vi "replaceTypeToken.vi"(8 "error in (no error)":errorcluster, 10 "Query In":string, 11 "Credit Transaction in":refnum<class "CreditTransaction.lvclass">) -> (0 "error out":errorcluster, 2 "Query Out":string, 3 "Credit Transaction out":refnum<class "CreditTransaction.lvclass">)   [LabVIEW 2018, in "CreditTransaction.lvclass"]
uses:
  CreditTransaction.lvclass
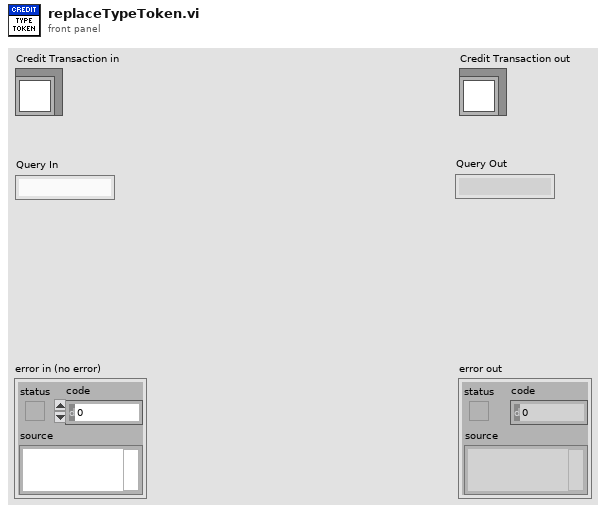
[diagram p1: front panel]
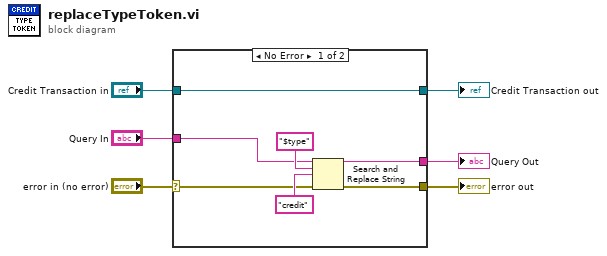
[diagram p0: block diagram]
diagram:
  n1 = case shown="No Error" "error in (no error)" {
    selector: "error in (no error)" -> [w7 w14]
    tunnel: [w9 w15] -> w5
    tunnel: "Query In" -> [w8 _]
    tunnel: "Credit Transaction in" -> [w9 w15]
    tunnel: [w13 w14] -> w4
    tunnel: [w12 _] -> w3
    frame No Error {
      n2 = Search and Replace String(input string=w8, search string="$type", replace string="credit" ("replace string (\"\")"), error in=w7) -> (result string=w12:string, error out=w13:errorcluster)  [unwired: 4 in, 2 out]
    }
    frame Error {
    }
  }
  "error out" <- w4
  "Credit Transaction out" <- w5
  "Query Out" <- w3
